vi "Settings Dialog.vi"(8 "error in (no error)":errorcluster, 11 "Settings in":T2) -> (0 "error out":errorcluster, 1 "Cancelled?":bool, 2 "UI Refresh Needed?":bool, 3 "Settings out":T2)   [LabVIEW 2018, in "Settings.lvlib"]
doc: "Dialog for selecting user specified settings."
uses:
  Settings.lvlib
  Settings.ctl
  Acquisition/Hardware Configuration.ctl
  Acquisition/Signal Type.ctl
  Logging/Logging Configuration.ctl
  <vilib>/Utility/xml.llb/Write to XML File(string).vi
  Acquisition/Acquisition.lvlib
  Logging/Logging.lvlib
panel:
  in  "Signal type":T1
  in  "Max writing time to file [min]":dbl
  in  "Test time zero run[s]":dbl
  in  "Test time [min]":dbl
  in  "Log File Offsite Path":path
  in  "Project code":string
  in  "Offsite storage?":bool
  in  "Log File Path":path
  in  "Cancel Button":bool
  in  "OK Button":bool
  # "Non visible portion of dialog (needed for connector pane)."
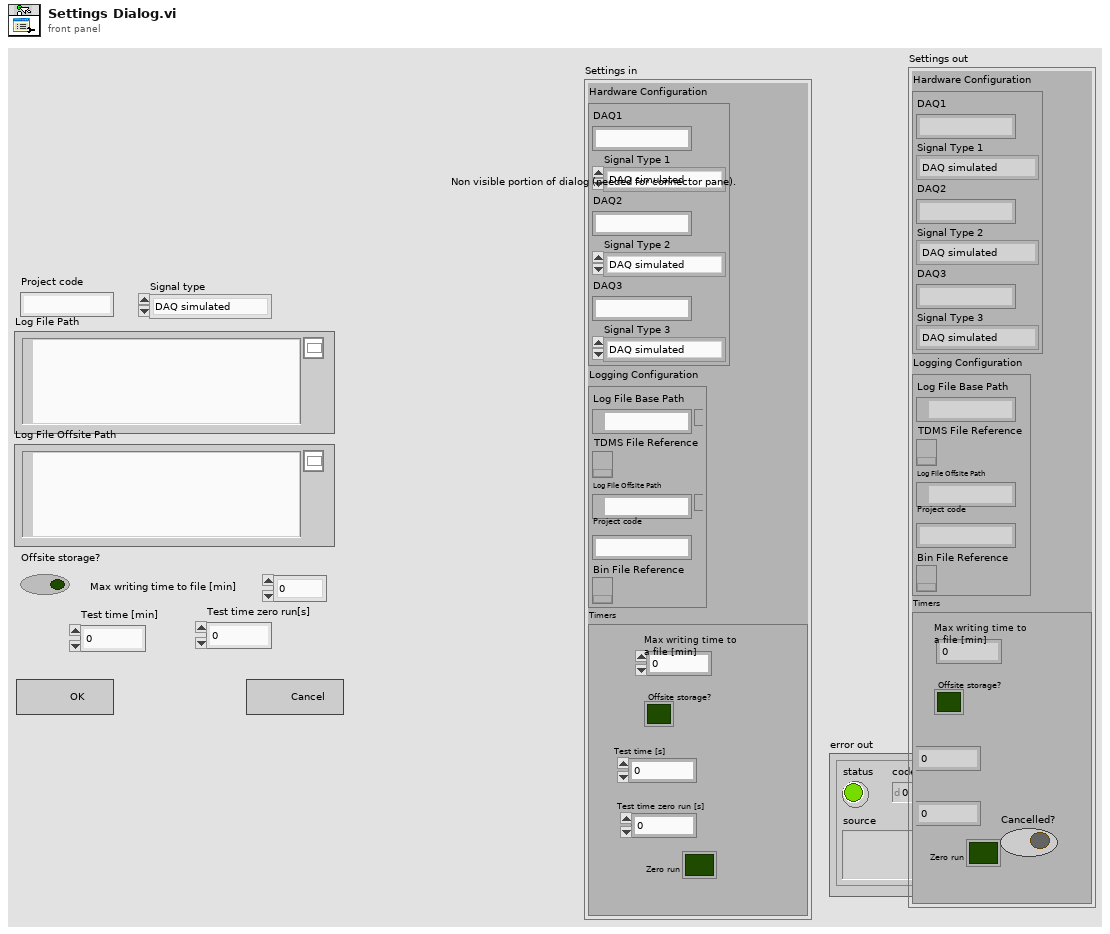
[diagram p1: front panel]
types:
  T1 = typedef "Acquisition.lvlib/Signal Type.ctl" = enum16{"DAQ simulated", "Sine and square wave", "Sine wave"}
  T2 = typedef "Settings.lvlib/Settings.ctl" = cluster{"Hardware Configuration":T3, "Logging Configuration":T4, "Timers":cluster{"Offsite storage?":bool, "Test time [s]":dbl, "Test time zero run [s] ":dbl, "Max writing time to a file [min]":dbl, "Zero run":bool}}
  T3 = typedef "Acquisition.lvlib/Hardware Configuration.ctl" = cluster{"DAQ1":string, "Signal Type 1":T1, "DAQ2":string, "Signal Type 2":T1, "DAQ3":string, "Signal Type 3":T1}
  T4 = typedef "Logging.lvlib/Logging Configuration.ctl" = cluster{"Log File Base Path":path, "TDMS File Reference":refnum<k34>, "Log File Offsite Path":path, "Project code":string, "Bin File Reference":refnum<k34>}
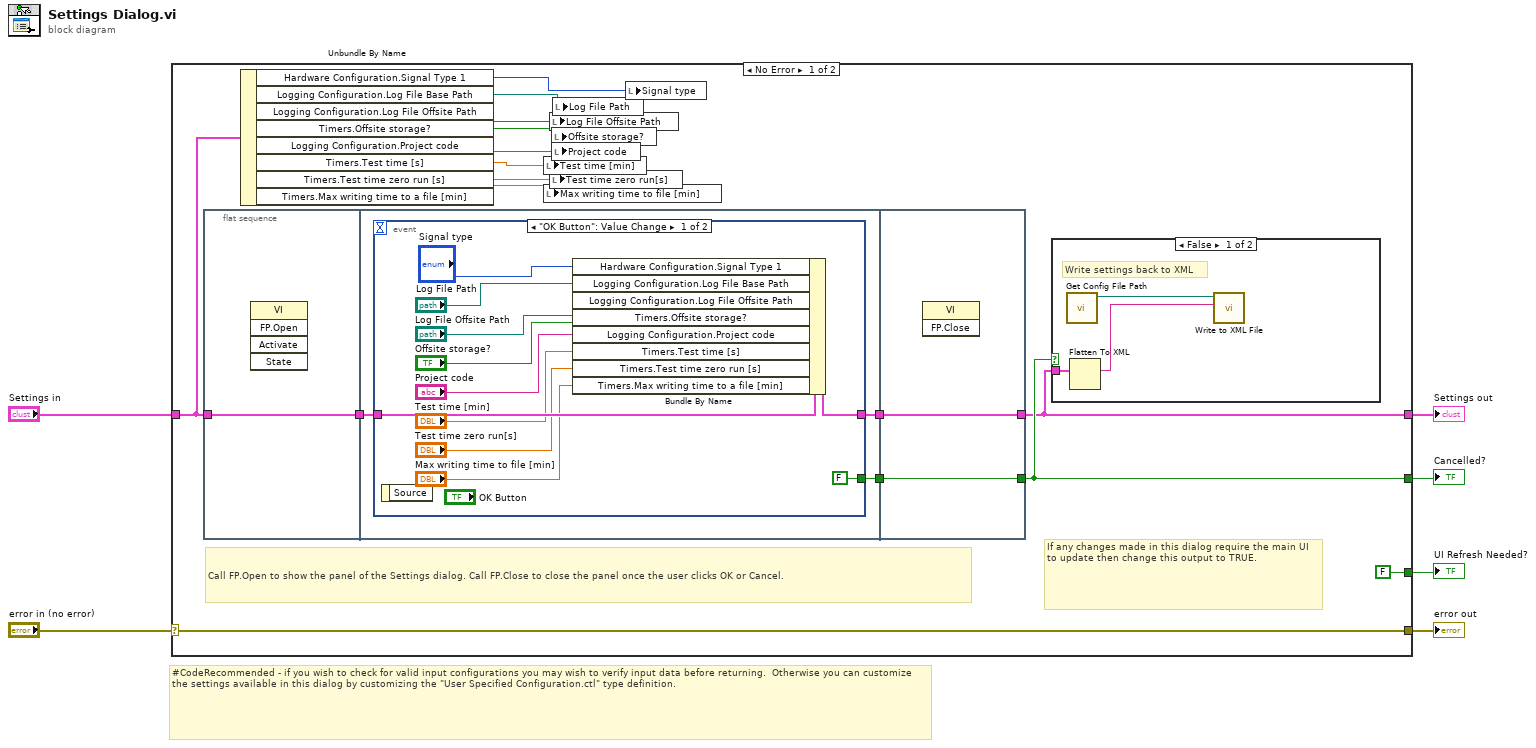
[diagram p0: block diagram]
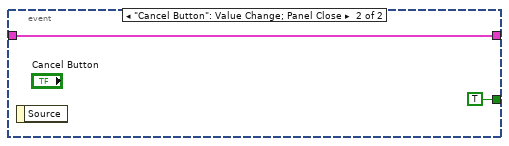
[diagram p2: hidden frame]
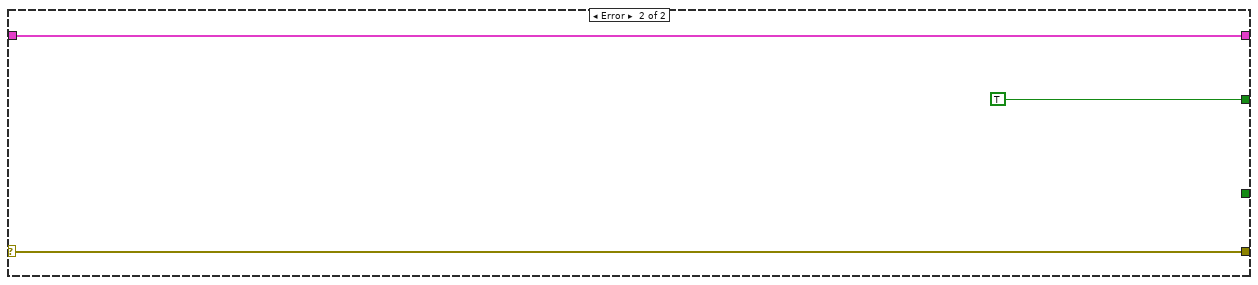
[diagram p4: hidden frame]
diagram:
  # "#CodeRecommended - if you wish to check for valid input configurations you may wish to verify input data before returning.  Otherwise you can customize the settings available in this dialog by customizing the \"User Specified Configuration.ctl\" type definition."
  n1 = case shown="No Error" "error in (no error)" {
    selector: "error in (no error)" -> [w22 w47]
    tunnel: [w22 w47] -> w5
    tunnel: "Settings in" -> [w18 w46]
    tunnel: [w19 w46] -> w3
    tunnel: [FALSE ("UI Refresh Needed?") _] -> w2
    tunnel: [w20 TRUE ("UI Refresh Needed?")] -> w1
    frame No Error {
      # "Call FP.Open to show the panel of the Settings dialog. Call FP.Close to close the panel once the user clicks OK or Cancel."
      # "If any changes made in this dialog require the main UI to update then change this output to TRUE."
      n2 = flat-sequence {
        tunnel: w18 -> [w23]
        tunnel: [w23] -> w16
        tunnel: w16 -> [w24]
        tunnel: [w26] -> w15
        tunnel: [w25] -> w14
        tunnel: [w40] -> w19
        tunnel: [w41] -> w20
        tunnel: w15 -> [w41]
        tunnel: w14 -> [w40]
        frame #0 {
          n3 = invoke class="VI" method="FP.Open"() -> ()  [unwired: 5 in, 5 out]
        }
        frame #1 {
          n4 = event shown="[0] \"OK Button\": Value Change" {
            selector: _ -> [_ _]
            dyn-events: _ -> [_ _]
            timeout: _ -> [_ _]
            tunnel: [w35 w39] -> w25
            tunnel: w24 -> [w36 w39]
            tunnel: [FALSE ("UI Refresh Needed?") TRUE ("UI Refresh Needed?")] -> w26
            event "OK Button": Value Change {
              n5 = event-data() -> ()  [unwired: 1 in, 1 out]
              n6 = Bundle By Name(cluster=w36, "Hardware Configuration.Signal Type 1"="Signal type", "Logging Configuration.Log File Base Path"="Log File Path", "Logging Configuration.Log File Offsite Path"="Log File Offsite Path", "Timers.Offsite storage?"="Offsite storage?", "Logging Configuration.Project code"="Project code", "Timers.Test time [s]"="Test time [min]", "Timers.Test time zero run [s]"="Test time zero run[s]", "Timers.Max writing time to a file [min]"="Max writing time to file [min]") -> (w35:T2)
            }
            event "Cancel Button": Value Change; Panel Close {
              n7 = event-data() -> ()  [unwired: 1 in, 1 out]
            }
          }
        }
        frame #2 {
          n8 = invoke class="VI" method="FP.Close"() -> ()  [unwired: 3 in, 3 out]
        }
      }
      n9 = Unbundle By Name(w18) -> ("Hardware Configuration.Signal Type 1"=w7:T1, "Logging Configuration.Log File Base Path"=w17:path, "Logging Configuration.Log File Offsite Path"=w13:path, "Timers.Offsite storage?"=w12:bool, "Logging Configuration.Project code"=w11:string, "Timers.Test time [s]"=w10:dbl, "Timers.Test time zero run [s]"=w9:dbl, "Timers.Max writing time to a file [min]"=w8:dbl)
      n10 = local write "Test time [min]"(w10) -> ()
      n11 = local write "Max writing time to file [min]"(w8) -> ()
      n12 = local write "Log File Offsite Path"(w13) -> ()
      n13 = local write "Test time zero run[s]"(w9) -> ()
      n14 = local write "Offsite storage?"(w12) -> ()
      n15 = local write "Project code"(w11) -> ()
      n16 = local write "Log File Path"(w17) -> ()
      n17 = local write "Signal type"(w7) -> ()
      n18 = case shown="False" w20 {
        tunnel: w19 -> [w43 _]
        frame False {
          # "Write settings back to XML"
          n19 = call "Get Config File Path.vi"() -> ("XML File Path"=w44:path)  [unwired: 10 in, 1 out]
          n20 = Flatten To XML(anything=w43) -> (xml string=w42:string)
          n21 = call-poly <vilib>:"Write to XML File.vi"("XML Input"=w42, "XML File Path"=w44) -> ()  [unwired: 7 in, 3 out]
        }
        frame True {
        }
      }
    }
    frame Error {
    }
  }
  "UI Refresh Needed?" <- w2
  "error out" <- w5
  "Settings out" <- w3
  "Cancelled?" <- w1
